vi "Read Reconnect.vi"(8 "error in (no error)":errorcluster, 11 "BaseDriver in":refnum<class "BaseDriver.lvclass">) -> (0 "error out":errorcluster, 2 "Reconnect?":bool=TRUE, 3 "BaseDriver out":refnum<class "BaseDriver.lvclass">)   [LabVIEW 2013, in "BaseDriver.lvclass"]
doc: "If TRUE, the driver will attempt to reconnect if it loses the connection to the remote host. If false, the driver will exit if connection is lost"
uses:
  BaseDriver.lvclass
  BaseDriver.lvclass/BaseDriver.ctl
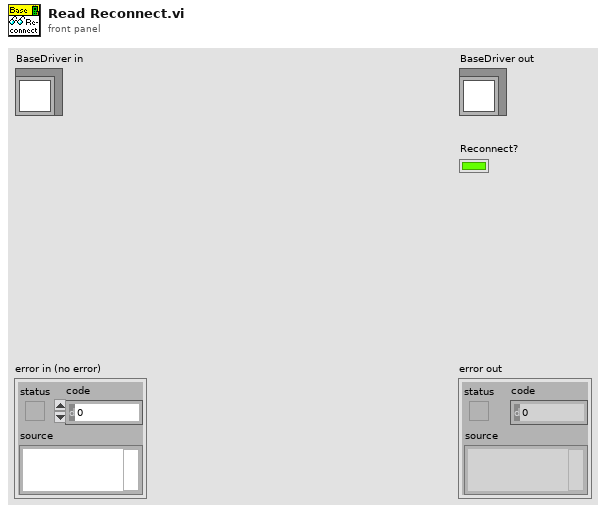
[diagram p1: front panel]
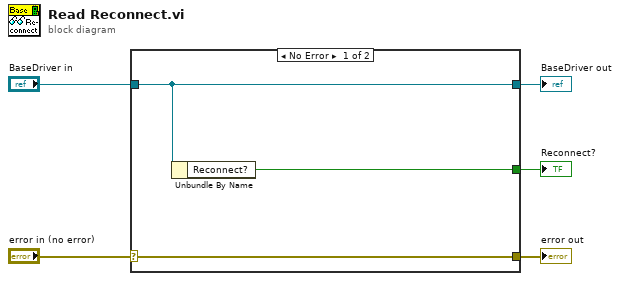
[diagram p0: block diagram]
diagram:
  n1 = case shown="No Error" "error in (no error)" {
    selector: "error in (no error)" -> [w8 w9]
    tunnel: [w8 w9] -> w4
    tunnel: [w7 w10] -> w2
    tunnel: "BaseDriver in" -> [w7 w10]
    tunnel: [w6 _] -> w1
    frame No Error {
      n2 = Unbundle By Name(w7) -> ("Reconnect?"=w6:bool)
    }
    frame Error {
    }
  }
  "error out" <- w4
  "BaseDriver out" <- w2
  "Reconnect?" <- w1
